vi "Serialisation Type.vi"(3 "MsgPackMessage in":refnum<class "WampMessage MsgPack.lvclass">) -> (1 "Serialisation Type":T1)   [LabVIEW 2020, in "wamplv.lvlib" / "WampMessage MsgPack.lvclass"]
uses:
  WampMessage MsgPack.lvclass
  WAMP Client/API/TypeDefs/Serialisation.ctl
  WampMessage MsgPack.lvclass/WampMessage MsgPack.ctl
  WAMP Client/WAMP Client.lvclass
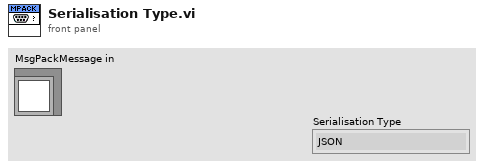
[diagram p1: front panel]
types:
  T1 = typedef "wamplv.lvlib/WAMP Client.lvclass/Serialisation.ctl" = enum16{"JSON", "MessagePack"}
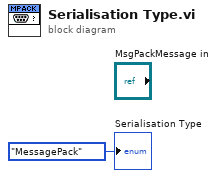
[diagram p0: block diagram]
diagram:
  "Serialisation Type" <- Serialisation."MessagePack" ("Serialisation Type")
